vi "PD500 - PWM test_v2.vi"(8 "Error In":errorcluster, 9 "Board Selector":T1, 10 "HMP VISA":refnum<visa-resource-name>, 11 "Control Board VISA":refnum<visa-resource-name>="ControlBoard") -> (0 "Error Out":errorcluster, 2 "Message OUT":string, 3 "Result (bool)":bool)   [LabVIEW 2022 SP3]
uses:
  Serial Board Com/Board Select.ctl
  HMP4000 Communication/HMP4040_ChannelControlAutomatic.ctl
  <vilib>/DAQmx/read.llb/DAQmx Read (Analog 1D Wfm NChan NSamp).vi
  <vilib>/DAQmx/miscellaneous.llb/DAQmx Fill In Error Info.vi
panel:
  out "Duty Cycle VISA Write":string[](array[string])
  out "Duty Cycles Measured":dbl[][](array[numeric])
  in  "Message IN":string=" "
  out "Analysis Leg":i32
  out "Waveforms":T2
  out "Active Leg":i32
  out "Result (color)":u32(colorbox)
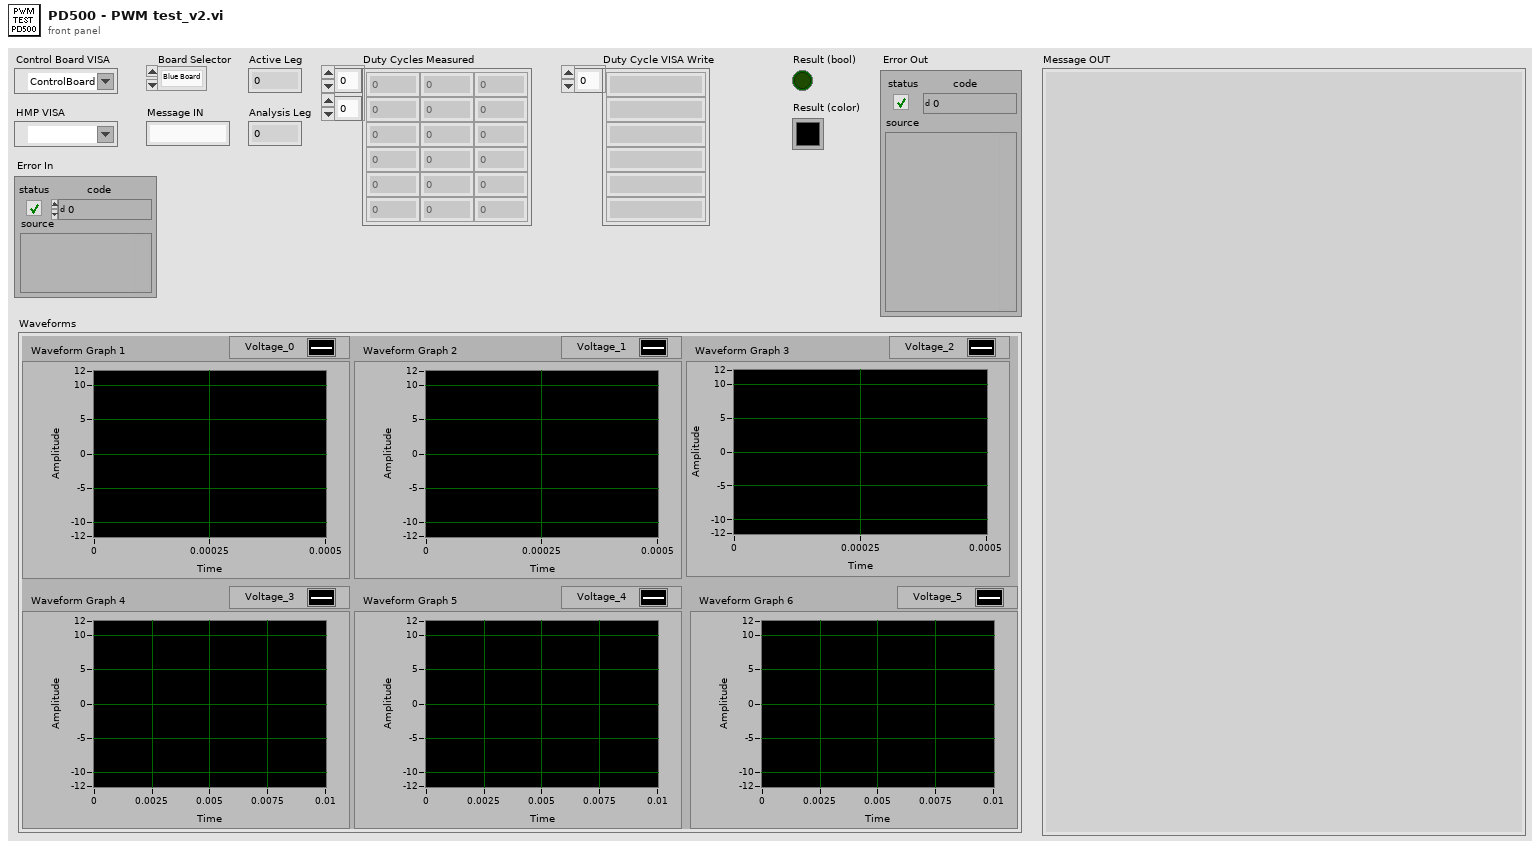
[diagram p1: front panel]
types:
  T1 = typedef "Board Select.ctl" = enum16{"Blue Board", "Green Board"}
  T2 = cluster{"Waveform Graph 1":waveform(dbl), "Waveform Graph 2":waveform(dbl), "Waveform Graph 3":waveform(dbl), "Waveform Graph 4":waveform(dbl), "Waveform Graph 5":waveform(dbl), "Waveform Graph 6":waveform(dbl)}
  T3 = typedef "HMP4040_ChannelControlAutomatic.ctl" = enum16{"Off", "Control Power", "HMP2020 Control + DC32V", "HMP2020 Control + DC8V", "HMP4040 Control + DC32V", "HMP4040 Control +DC8V", "HMP4040 Ch2 24V 4A"}
  T4 = cluster{"data[0]":waveform(dbl), "data[1]":waveform(dbl), "data[2]":waveform(dbl), "data[3]":waveform(dbl), "data[4]":waveform(dbl), "data[5]":waveform(dbl)}
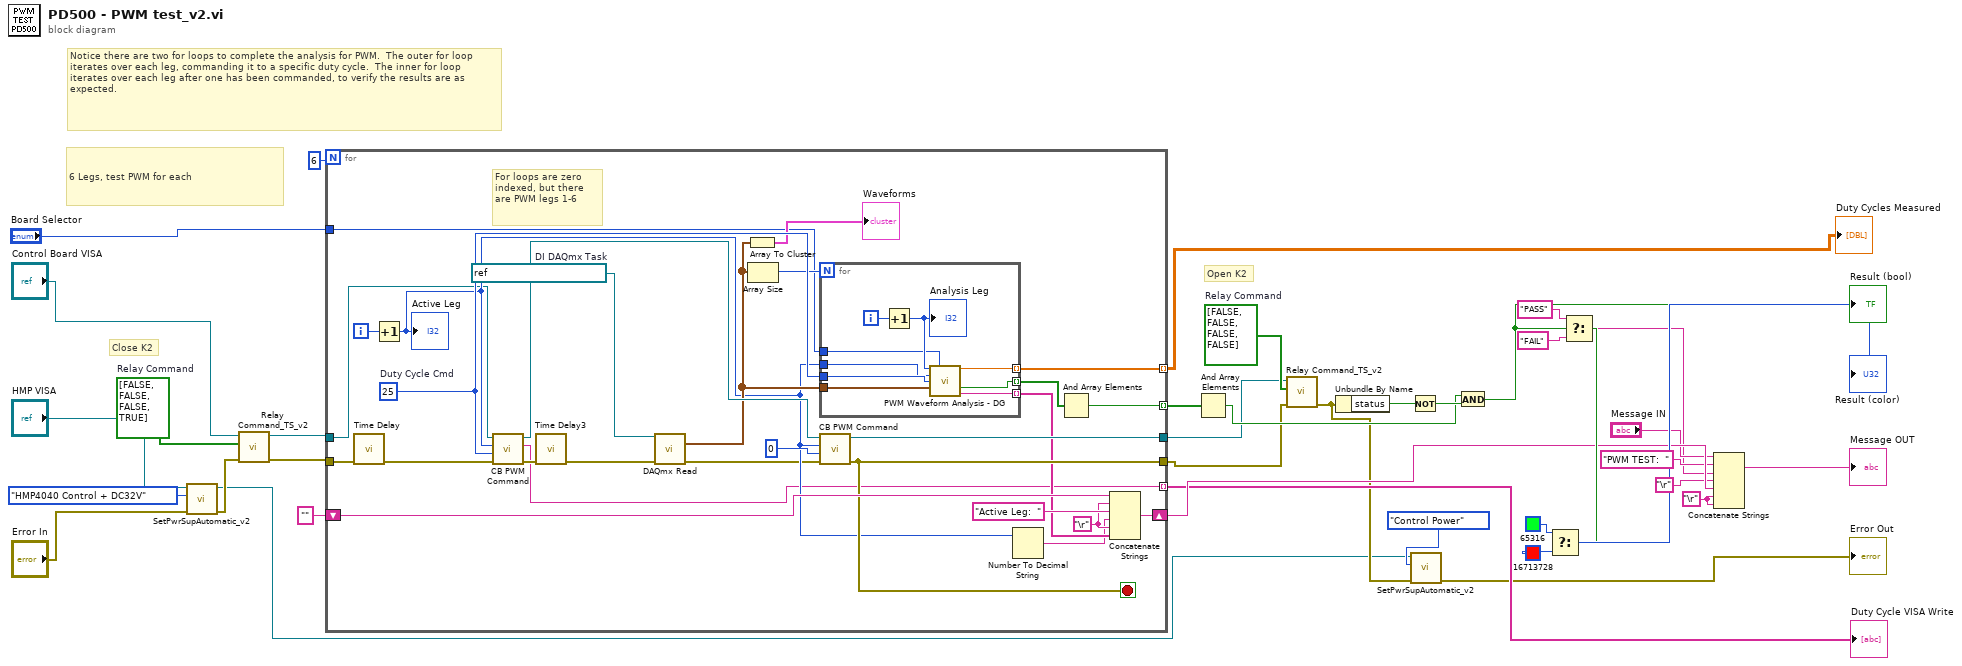
[diagram p0: block diagram]
diagram:
  w13 = bool[] [FALSE, FALSE, FALSE, TRUE]  # Relay Command
  w7 = bool[] [FALSE, FALSE, FALSE, FALSE]  # Relay Command
  w26 = "\r"
  # "Close K2"
  # "Open K2"
  # "Notice there are two for loops to complete the analysis for PWM.  The outer for loop iterates over each leg, commanding it to a specific duty cycle.  The inner for loop iterates over each leg after one has been commanded, to verify the results are as expected."
  # "6 Legs, test PWM for each"
  n1 = call "SetPwrSupAutomatic_v2.vi"("error in (no error)"="Error In", "Enum"=HMP4040_ChannelControlAutomatic."HMP4040 Control + DC32V", "HMP VISA"="HMP VISA") -> ("error out"=w11:errorcluster, "HMP VISA Out"=w4:refnum<visa-resource-name>)  [unwired: 7 in]
  n2 = call "Relay Command_TS_v2.vi"("error in (no error)"=w11, "Relay Command"=w13, "Control Board VISA"="Control Board VISA") -> ("error out"=w16:errorcluster, "VISA Refnum out"=w17:refnum<visa-resource-name>)  [unwired: 7 in]
  n3 = for {
    N: 6 -> [_]
    tunnel: [w65] -> w37 mode=indexing
    shift-right: [w63] -> w24
    shift-left: "" -> [w62]
    tunnel: [w57] -> w18
    tunnel: [w52] -> w2
    tunnel: w16 -> [w40]
    tunnel: w17 -> [w46]
    tunnel: [w43] -> w15 mode=indexing
    tunnel: [w42] -> w14 mode=indexing
    tunnel: "Board Selector" -> [w41]
    i -> [w58]
    stop <- w57 stop-if-true
    w48 = "\r"
    w59 = 25  # Duty Cycle Cmd
    w64 = refnum<k21> "FTS2_PWMInput_DG"  # DI DAQmx Task
    # "For loops are zero indexed, but there are PWM legs 1-6"
    n4 = call "Time Delay"("error in (no error)"=w40) -> ("error out"=w39:errorcluster)  [unwired: 10 in]
    n5 = Increment(x=w58) -> (x+1=w50:i32)
    "Active Leg" <- w50
    n6 = call "CB PWM Command.vi"("error in (no error)"=w39, "Duty Cycle"=w59, "Leg"=w50, "VISA Refnum in"=w46) -> ("error out"=w45:errorcluster, "read buffer"=w42:string, "VISA Refnum out"=w60:refnum<visa-resource-name>)  [unwired: 5 in]
    n7 = call "Time Delay3"("error in (no error)"=w45) -> ("error out"=w44:errorcluster)  [unwired: 10 in]
    n8 = call-poly <vilib>:"DAQmx Read.vi"("task/channels in"=w64, "error in"=w44) -> ("data"=w53:waveform(dbl)[], "error out"=w38:errorcluster)  [unwired: 11 in, 1 out]
    n9 = Array To Cluster(array=w53) -> (cluster=→"Waveforms":T4)
    n10 = Array Size(array=w53) -> (size(s)=w54:i32)
    n11 = for {
      N: w54 -> [_]
      tunnel: w59 -> [w74]
      tunnel: w53 -> [w73]
      tunnel: w50 -> [w72]
      tunnel: [w69] -> w55 mode=indexing
      tunnel: [w68] -> w49 mode=indexing
      tunnel: [w67] -> w43 mode=indexing
      tunnel: w41 -> [w66]
      i -> [w71]
      n12 = Increment(x=w71) -> (x+1=w70:i32)
      "Analysis Leg" <- w70
      n13 = call "PWM Waveform Analysis - DG.vi"("Analysis Leg"=w70, "Board Selector"=w66, "Active Leg"=w72, "Duty Cycle"=w74, "Waveform"=w73) -> ("Active Leg Actual Duty"=w67:dbl, "Result (Boolean)"=w69:bool, "Message"=w68:string)  [unwired: 8 in]
    }
    n14 = call "CB PWM Command.vi"("error in (no error)"=w38, "Duty Cycle"=0, "Leg"=w50, "VISA Refnum in"=w60) -> ("error out"=w57:errorcluster, "VISA Refnum out"=w52:refnum<visa-resource-name>)  [unwired: 5 in, 1 out]
    n15 = Number To Decimal String(number=w50) -> (decimal integer string=w47:string)  [unwired: 1 in]
    n16 = And Array Elements(Boolean array=w55) -> (logical AND=w65:bool)
    n17 = Concatenate Strings(w62, w48, "Active Leg:  ", w47, w48, w49) -> (w63:string)
  }
  "Duty Cycles Measured" <- w15
  "Duty Cycle VISA Write" <- w14
  n18 = And Array Elements(Boolean array=w37) -> (logical AND=w27:bool)
  n19 = call "Relay Command_TS_v2.vi"("error in (no error)"=w18, "Relay Command"=w7, "Control Board VISA"=w2) -> ("error out"=w10:errorcluster)  [unwired: 7 in, 1 out]
  n20 = Unbundle By Name(w10) -> ("status"=w30:bool)
  n21 = Not(x=w30) -> (.not. x?=w29:bool)
  n22 = call "SetPwrSupAutomatic_v2.vi"("error in (no error)"=w10, "Enum"=HMP4040_ChannelControlAutomatic."Control Power", "HMP VISA"=w4) -> ("error out"=→"Error Out":errorcluster)  [unwired: 7 in, 1 out]
  n23 = And(x=w27, y=w29) -> (x .and. y?=w28:bool)
  "Result (bool)" <- w28
  n24 = Select(t=u32 65316 ("Result (color)"), s=w28, f=u32 16713728 ("Result (color)")) -> (s? t:f=→"Result (color)":u32)
  n25 = Select(t="PASS", s=w28, f="FAIL") -> (s? t:f=w19:string)
  n26 = Concatenate Strings("Message IN", "PWM TEST:  ", w19, "\r", w24, w26, w26) -> (→"Message OUT":string)
